vi "solar_voy Get Bits (Variant).vi"(6 "Suppress Errors? (T)":bool=TRUE, 7 "Endian (BIG)":enum8{"BIG", "LITTLE"}(ring), 8 "error in (no error)":errorcluster, 10 "COSMOS Data":string, 11 "ITEMS in":T1[](array[typedef])) -> (0 "error out":errorcluster, 1 "Item Values (LV Flattened Value)":string[](array[string]), 2 "Item Values":variant[](array[variant]), 3 "ITEMS out":T1[](array[typedef]))   [LabVIEW 2018]
doc: "This unpacks the COSMOS Data into an array of items and variant array."
uses:
  solar_voy_def/solar_voy_def_ctl MODIFIERS LIMITS.ctl
  solar_voy_def/solar_voy_def_ctl MODIFIERS UNITS.ctl
  solar_voy_def/solar_voy_def_ctl MODIFIERS STATE.ctl
  solar_voy_def/solar_voy_def_ctl MODIFIERS CONVERSION.ctl
  solar_voy_def/solar_voy_def_ctl MODIFIERS.ctl
  solar_voy_def/solar_voy_def_ctl ITEM TYPE.ctl
  type/solar_type Item Type.ctl
  solar_voy_def/solar_voy_def_ctl ITEM.ctl
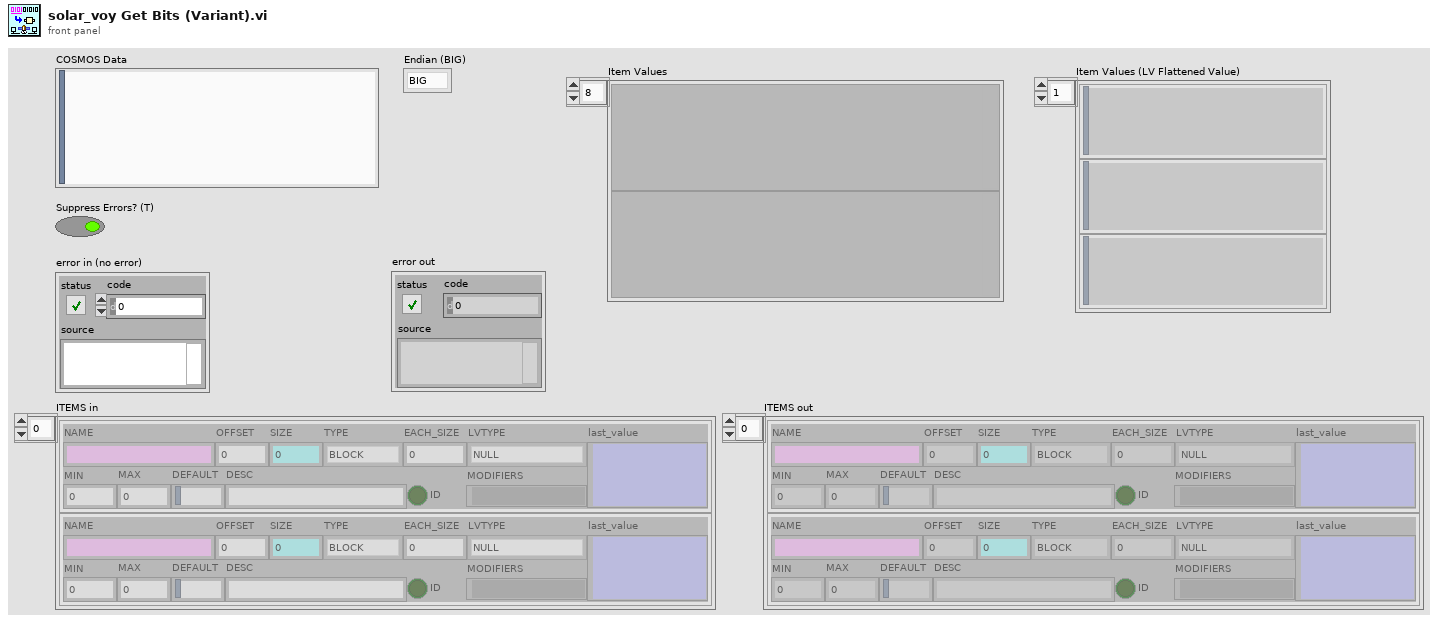
[diagram p1: front panel]
types:
  T1 = typedef "solar_voy_def_ctl ITEM.ctl" = cluster{"NAME":string, "OFFSET":i32, "SIZE":i32, "TYPE":T2, "EACH_SIZE":i32, "LVTYPE":T3, "MIN":dbl, "MAX":dbl, "DEFAULT":string, "DESC":string, "ID":bool, "MODIFIERS":variant, "last_value":variant}
  T2 = typedef "solar_voy_def_ctl ITEM TYPE.ctl" = enum8{"BLOCK", "INT", "UINT", "FLOAT", "STRING"}
  T3 = typedef "solar_type Item Type.ctl" = enum16{"NULL", "UNKNOWN", "CLUSTER", "I8", "I16", "I32", "I64", "U8", "U16", "U32", "U64", "U8_ENUM", "U16_ENUM", "U32_ENUM", "SGL", "DBL", "BOOLEAN", "STRING", "PATH", "VISA", "TAG", "TIME", "I8_1D", "I16_1D", "I32_1D", "I64_1D", "U8_1D", "U16_1D", "U32_1D", "U64_1D", "U8_ENUM_1D", "U16_ENUM_1D", "U32_ENUM_1D", "SGL_1D", "DBL_1D", "BOOLEAN_1D", "STRING_1D", "PATH_1D", "VISA_1D", "TAG_1D", "TIME_1D", "I8_2D", "I16_2D", "I32_2D", "I64_2D", "U8_2D", "U16_2D", "U32_2D", "U64_2D", "U8_ENUM_2D", "U16_ENUM_2D", "U32_ENUM_2D", "SGL_2D", "DBL_2D", "BOOLEAN_2D", "STRING_2D", "PATH_2D", "VISA_2D", "TAG_2D", "TIME_2D"}
  T4 = typedef "solar_voy_def_ctl MODIFIERS.ctl" = cluster{"LIMITS":T5, "UNITS":T6, "STATES":T7[], "CONVERSION":T8, "FORMAT":string, "REQUIRED":bool, "META":string[][]}
  T5 = typedef "solar_voy_def_ctl MODIFIERS LIMITS.ctl" = cluster{"NAME":string, "PERSIST":i32, "EN":bool, "RED_LO":dbl, "YEL_LO":dbl, "YEL_HI":dbl, "RED_HI":dbl, "GRN_LO":dbl, "GRN_HI":dbl, "FILENAME":string, "ARGS":string}
  T6 = typedef "solar_voy_def_ctl MODIFIERS UNITS.ctl" = cluster{"FULL":string, "ABV":string}
  T7 = typedef "solar_voy_def_ctl MODIFIERS STATE.ctl" = cluster{"KEY":string, "VALUE":string, "COLOR":string, "DESC":string, "HZRD":bool}
  T8 = typedef "solar_voy_def_ctl MODIFIERS CONVERSION.ctl" = cluster{"GENERIC":string, "FILENAME":string, "ARGS":string, "POLYS":cluster{"SEG":bool, "POLY":dbl[]}[]}
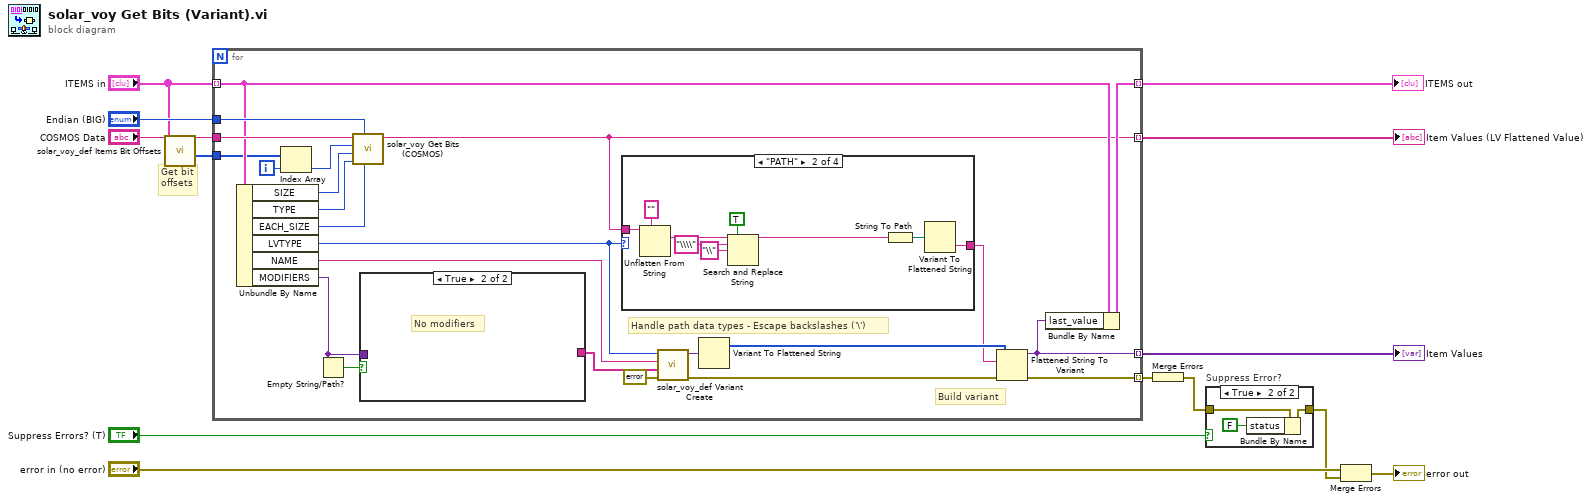
[diagram p0: block diagram]
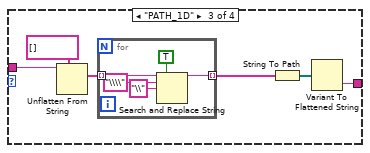
[diagram p3: hidden frame]
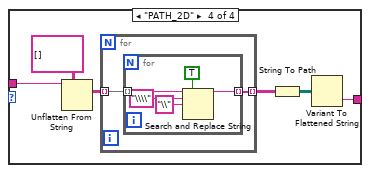
[diagram p4: hidden frame]
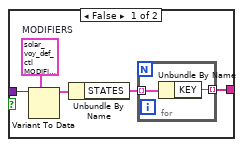
[diagram p5: hidden frame]
diagram:
  # "Get bit\noffsets"
  n1 = call "solar_voy_def Items Bit Offsets.vi"("ITEMS in"="ITEMS in") -> ("Bit Offsets"=w1:i32[])  [unwired: 9 in, 1 out]
  n2 = for {
    tunnel: "Endian (BIG)" -> [w35]
    tunnel: "COSMOS Data" -> [w36]
    tunnel: [w24] -> w11 mode=indexing
    tunnel: [w26] -> w7 mode=indexing
    tunnel: [w15] -> w8 mode=indexing
    tunnel: "ITEMS in" -> [w22] mode=indexing
    tunnel: [w23] -> w3 mode=indexing
    tunnel: w1 -> [w21]
    i -> [w19]
    # "Handle path data types - Escape backslashes ('\\')"
    # "Build variant"
    n3 = Unbundle By Name(w22) -> ("SIZE"=w34:i32, "TYPE"=w33:T2, "EACH_SIZE"=w32:i32, "LVTYPE"=w16:T3, "NAME"=w25:string, "MODIFIERS"=w18:variant)
    n4 = Index Array(array=w21, index=w19) -> (element=w20:i32)
    n5 = Empty String/Path?(string/path=w18) -> (empty?=w17:bool)
    n6 = call "solar_voy Get Bits (COSMOS).vi"("Bit Element Size (Array only)"=w32, "Endian (BIG)"=w35, "COSMOS TYPE"=w33, "Bit Size"=w34, "Bit Offset"=w20, "COSMOS Data"=w36) -> ("LabVIEW Flattened Value"=w15:string)  [unwired: 4 in, 1 out]
    n7 = case shown="True" w17 {
      tunnel: [w75 _] -> w31
      tunnel: w18 -> [w71 _]
      frame False {
        w74 = T4 {"LIMITS"={"NAME"="", "PERSIST"=0, "EN"=FALSE, "RED_LO"=0.0, "YEL_LO"=0.0, "YEL_HI"=0.0, "RED_HI"=0.0, "GRN_LO"=0.0, "GRN_HI"=0.0, "FILENAME"="", "ARGS"=""}, "UNITS"={"FULL"="", "ABV"=""}, "STATES"=[], "CONVERSION"={"GENERIC"="", "FILENAME"="", "ARGS"="", "POLYS"=[]}, "FORMAT"="", "REQUIRED"=FALSE, "META"=[]}  # MODIFIERS
        n8 = Variant To Data(type=w74, Variant=w71) -> (data=w73:T4)  [unwired: 1 in, 1 out]
        n9 = Unbundle By Name(w73) -> ("STATES"=w72:T7[])
        n10 = for {
          tunnel: w72 -> [w77] mode=indexing
          tunnel: [w76] -> w75 mode=indexing
          n11 = Unbundle By Name(w77) -> ("KEY"=w76:string)
        }
      }
      frame True {
        # "No modifiers"
      }
    }
    n12 = case shown="\"PATH\"" w16 {
      tunnel: w15 -> [w37 w46 w52 w63]
      tunnel: [w37 w43 w49 w60] -> w14
      frame Default {
      }
      frame "PATH" {
        n13 = Unflatten From String(type="", binary string=w46) -> (value=w39:string)  [unwired: 3 in, 2 out]
        n14 = Search and Replace String(replace all?=TRUE ("replace all? (F)"), input string=w39, search string="\\\\", replace string="\\" ("search string")) -> (result string=w38:string)  [unwired: 4 in, 3 out]
        n15 = String To Path(string=w38) -> (path=w44:path)
        n16 = Variant To Flattened String(Variant=w44) -> (data string=w43:string)  [unwired: 1 out]
      }
      frame "PATH_1D" {
        n17 = Unflatten From String(type=string[] [], binary string=w52) -> (value=w48:string[])  [unwired: 3 in, 2 out]
        n18 = for {
          tunnel: w48 -> [w54] mode=indexing
          tunnel: [w53] -> w47 mode=indexing
          n19 = Search and Replace String(replace all?=TRUE ("replace all? (F)"), input string=w54, search string="\\\\", replace string="\\" ("search string")) -> (result string=w53:string)  [unwired: 4 in, 3 out]
        }
        n20 = String To Path(string=w47) -> (path=w50:path[])
        n21 = Variant To Flattened String(Variant=w50) -> (data string=w49:string)  [unwired: 1 out]
      }
      frame "PATH_2D" {
        n22 = Unflatten From String(type=string[][] [], binary string=w63) -> (value=w59:string[][])  [unwired: 3 in, 2 out]
        n23 = for {
          tunnel: w59 -> [w65] mode=indexing
          tunnel: [w64] -> w58 mode=indexing
          n24 = for {
            tunnel: w65 -> [w67] mode=indexing
            tunnel: [w66] -> w64 mode=indexing
            n25 = Search and Replace String(replace all?=TRUE ("replace all? (F)"), input string=w67, search string="\\\\", replace string="\\" ("search string")) -> (result string=w66:string)  [unwired: 4 in, 3 out]
          }
        }
        n26 = String To Path(string=w58) -> (path=w61:path[][])
        n27 = Variant To Flattened String(Variant=w61) -> (data string=w60:string)  [unwired: 1 out]
      }
    }
    n28 = call "solar_voy_def Variant Create.vi"("error in (no error)"=errorcluster {"status"=FALSE, "code"=0, "source"=""} ("error out"), "Enum Names"=w31, "Name"=w25, "LVTYPE"=w16) -> ("error out"=w29:errorcluster, "Variant"=w28:variant)  [unwired: 6 in]
    n29 = Variant To Flattened String(Variant=w28) -> (1:w30:i16[])  [unwired: 1 out]
    n30 = Flattened String To Variant(4:w29, 6:w14, 7:w30) -> (0:w26:errorcluster, 3:w24:variant)
    n31 = Bundle By Name(cluster=w22, "last_value"=w24) -> (w23:T1)
  }
  "Item Values" <- w11
  "Item Values (LV Flattened Value)" <- w8
  "ITEMS out" <- w3
  n32 = Merge Errors(w7) -> (w2:errorcluster)
  n33 = case "Suppress Error?" shown="True" "Suppress Errors? (T)" {
    tunnel: w2 -> [w78 w81]
    tunnel: [w78 w80] -> w6
    frame False {
    }
    frame True {
      n34 = Bundle By Name(cluster=w81, "status"=FALSE) -> (w80:errorcluster)
    }
  }
  n35 = Merge Errors("error in (no error)", w6) -> (→"error out":errorcluster)
